vi "Max&Min_withThr_subVI.vi"(5 "Soglia":dbl, 6 "magnitude":cluster{"f0":dbl, "df":dbl, "magnitude":dbl[]} {"magnitude" format="%.2p"; "f0" format="%0.2p"; "df" format="%0.2p"}) -> (0 "Ampiezza min":string, 1 "freq ad ampiezza min":string, 2 "Ampiezza max":string, 3 "freq ad ampiezza max":string, 4 "OverThr":bool)   [LabVIEW 2018]
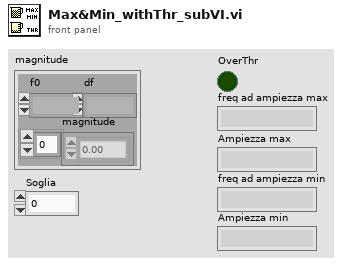
[diagram p1: front panel]
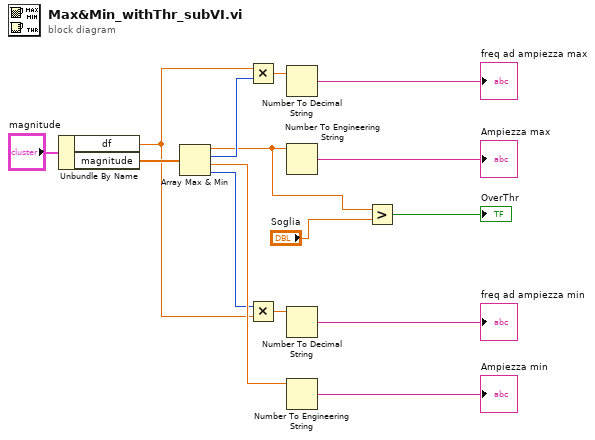
[diagram p0: block diagram]
diagram:
  n1 = Unbundle By Name("magnitude") -> ("df"=w9:dbl, "magnitude"=w15:dbl[])
  n2 = Array Max & Min(array=w15) -> (max value=w7:dbl, max index (indices)=w12:i32, min value=w11:dbl, min index (indices)=w10:i32)
  n3 = Multiply(x=w9, y=w12) -> (x*y=w13:dbl)
  n4 = Multiply(x=w10, y=w9) -> (x*y=w8:dbl)
  n5 = Number To Decimal String(number=w13) -> (decimal integer string=→"freq ad ampiezza max":string)  [unwired: 1 in]
  n6 = Number To Engineering String(4:w7) -> (0:→"Ampiezza max":string)  [unwired: 3 in]
  n7 = Number To Decimal String(number=w8) -> (decimal integer string=→"freq ad ampiezza min":string)  [unwired: 1 in]
  n8 = Number To Engineering String(4:w11) -> (0:→"Ampiezza min":string)  [unwired: 3 in]
  n9 = Greater?(x=w7, y="Soglia") -> (0:→"OverThr":bool)
